vi "FW_readFiles.vi"(4 "frame_offset":i32, 6 "amount_frames":u32, 7 "Decimate_frameRate":i32, 8 "error in (no error)":errorcluster, 10 "path(dir/img)":path[](array[path]), 11 "JPG/AVI (F:JPG)":bool) -> (0 "error out":errorcluster, 2 "image_path_array_out":path[](array[path]), 3 "image_array_out":T1[](array[typedef]), 5 "root folder":path)   [LabVIEW 2021, in "Framework_lib.lvlib"]
uses:
  QMH/Framework_lib.lvlib
  <vilib>/vision/Image Controls.llb/IMAQ Image.ctl
  <vilib>/vision/Avi.llb/IMAQ AVI2 Codec Path.ctl
panel:
  out "frame #":i32
  out "elapsed(ms)":u32
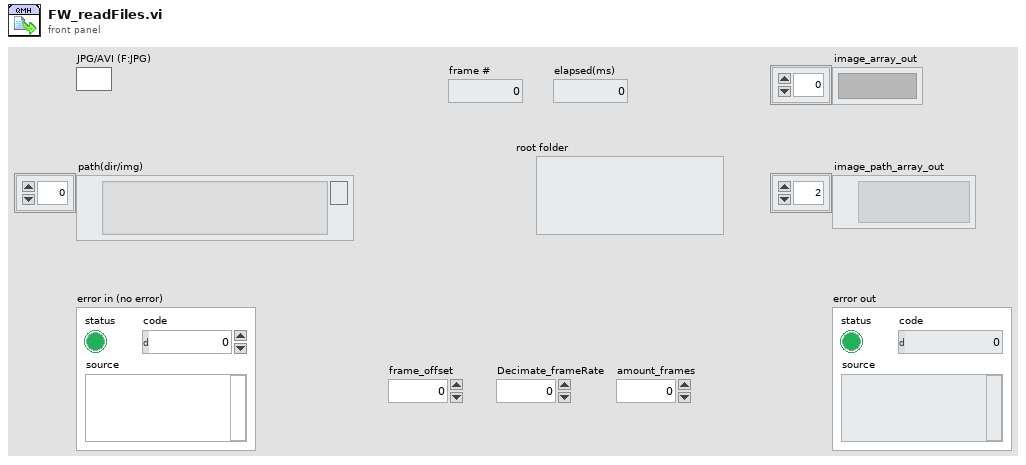
[diagram p1: front panel]
types:
  T1 = typedef "IMAQ Image.ctl" = refnum<image>
  T2 = typedef "IMAQ AVI2 Codec Path.ctl" = u32
  T3 = typedef "IMAQ AVI2 Refnum.ctl" = refnum<k20>
  T4 = typedef "Image Type" = u32
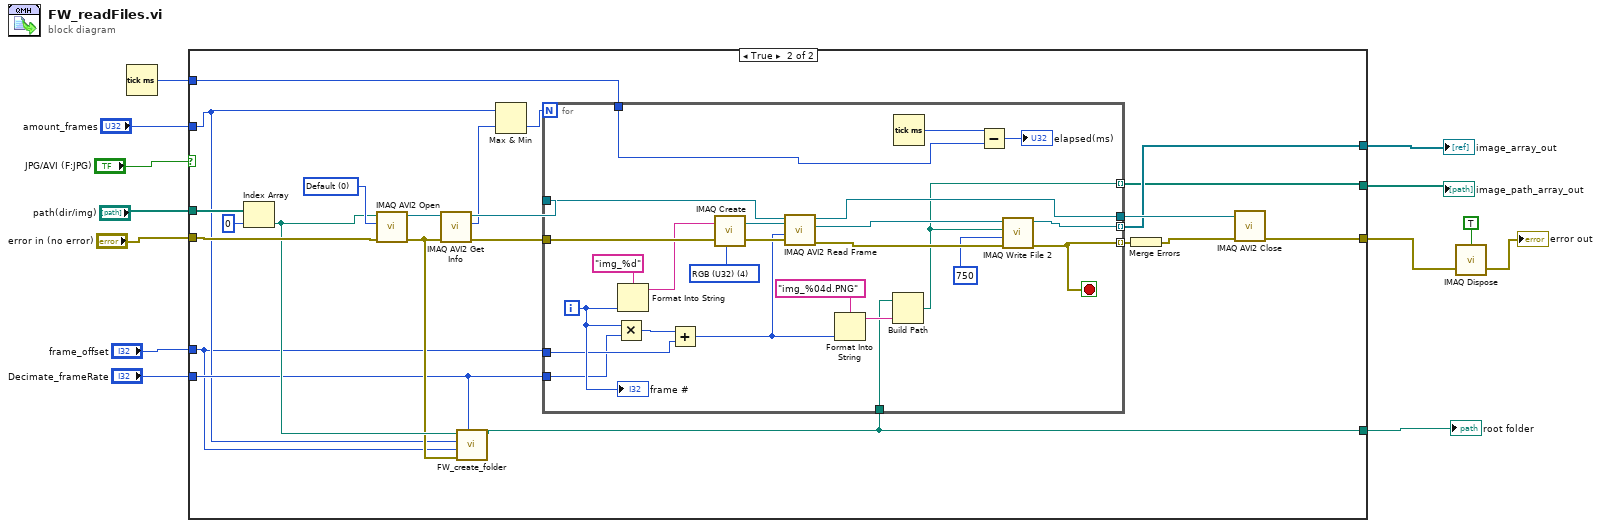
[diagram p0: block diagram]
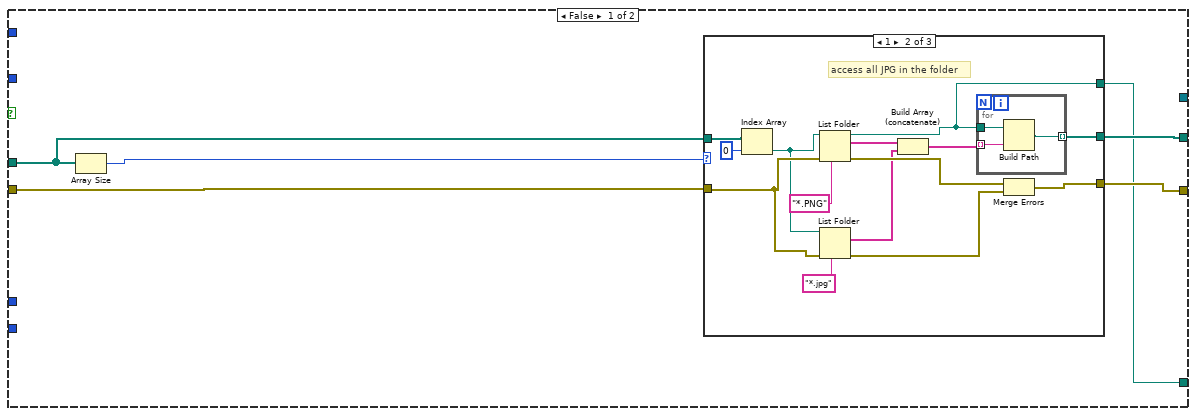
[diagram p2: hidden frame]
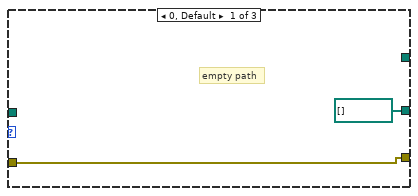
[diagram p3: hidden frame]
diagram:
  n1 = Tick Count (ms)() -> (millisecond timer value=w4:u32)
  n2 = case shown="True" "JPG/AVI (F:JPG)" {
    tunnel: "path(dir/img)" -> [w18 w61]
    tunnel: "error in (no error)" -> [w17 w59]
    tunnel: [w16 w58] -> w13
    tunnel: [w15 w46] -> w9
    tunnel: [_ w51] -> w8
    tunnel: "amount_frames" -> [_ w42]
    tunnel: "frame_offset" -> [_ w41]
    tunnel: "Decimate_frameRate" -> [_ w45]
    tunnel: w4 -> [_ w44]
    tunnel: [w14 w43] -> w3
    frame False {
      n3 = Array Size(array=w18) -> (size(s)=w19:i32)
      n4 = case shown="1" w19 {
        tunnel: w18 -> [_ w35 w40]
        tunnel: w17 -> [w20 w27 w39]
        tunnel: [w20 w26 w39] -> w16
        tunnel: [path[] [] w30 w40] -> w15
        tunnel: [_ w29 _] -> w14
        frame 0, Default {
          # "empty path"
        }
        frame 1 {
          # "access all JPG in the folder"
          n5 = Index Array(array=w35, index=0) -> (element=w22:path)
          n6 = List Folder(path=w22, pattern="*.PNG", error in=w27) -> (path out=w29:path, filenames=w31:string[], error out=w32:errorcluster)  [unwired: 1 in, 1 out]
          n7 = List Folder(path=w22, pattern="*.jpg", error in=w27) -> (filenames=w23:string[], error out=w25:errorcluster)  [unwired: 1 in, 2 out]
          n8 = Build Array (concatenate)(w31, w23) -> (w24:string[])
          n9 = for {
            tunnel: w29 -> [w38]
            tunnel: w24 -> [w37] mode=indexing
            tunnel: [w36] -> w30 mode=indexing
            n10 = Build Path(base path=w38, name or relative path=w37) -> (appended path=w36:path)
          }
          n11 = Merge Errors(w32, w25) -> (w26:errorcluster)
        }
        frame 2.. {
          # "read each file (must be JPG)"
        }
      }
    }
    frame True {
      w62 = T2 0 items=["Default", "System", "Built in Vision"] ("Codec Source")
      n12 = Index Array(array=w61, index=0) -> (element=w48:path)
      n13 = call "IMAQ AVI2 Open"("error in (no error)"=w59, "Codec Source"=w62, "AVI File Path"=w48) -> ("error out"=w47:errorcluster, "AVI Refnum"=w57:T3)  [unwired: 7 in]
      n14 = call "IMAQ AVI2 Get Info"("error in (no error)"=w47, "AVI Refnum"=w57) -> ("error out"=w56:errorcluster, "Number of Frames"=w50:u32, "AVI Refnum (duplicate)"=w55:T3)  [unwired: 5 in, 2 out]
      n15 = call "FW_create_folder.vi"("Decimate_frameRate"=w45, "error in (no error)"=w47, "frame_offset"=w41, "amount_frames"=w42, "Path"=w48) -> ("created path"=w43:path)  [unwired: 5 in, 1 out]
      n16 = Max & Min(x=w42, y=w50) -> (min(x,y)=w49:u32)  [unwired: 1 out]
      n17 = for {
        N: w49 -> [_]
        tunnel: w56 -> [w87]
        tunnel: w55 -> [w83]
        tunnel: [w77] -> w54 mode=indexing
        tunnel: [w81] -> w53
        tunnel: [w75] -> w51 mode=indexing
        tunnel: w41 -> [w74]
        tunnel: w43 -> [w71]
        tunnel: [w70] -> w46 mode=indexing
        tunnel: w45 -> [w68]
        tunnel: w44 -> [w64]
        i -> [w78]
        stop <- w77 stop-if-true
        w86 = T4 4 items=["Grayscale (U8)", "Grayscale (I16)", "Grayscale (SGL)", "Complex (CSG)", "RGB (U32)", "HSL (U32)", "RGB (U64)", "Grayscale (U16)"] ("Image Type")
        n18 = Multiply(x=w78, y=w68) -> (x*y=w69:i32)
        n19 = Format Into String(format string="img_%d", w78) -> (resulting string=w80:string)  [unwired: 2 in, 1 out]
        n20 = Add(x=w69, y=w74) -> (x+y=w67:i32)
        n21 = call "IMAQ Create"("Image Name"=w80, "Image Type"=w86, "error in (no error)"=w87) -> ("New Image"=w84:T1, "error out"=w85:errorcluster)  [unwired: 2 in]
        n22 = call "IMAQ AVI2 Read Frame"("error in (no error)"=w85, "Frame Number"=w67, "Image"=w84, "AVI Refnum"=w83) -> ("error out"=w82:errorcluster, "Image Out"=w76:T1, "AVI Refnum (duplicate)"=w81:T3)  [unwired: 5 in]
        n23 = Format Into String(format string="img_%04d.PNG", w67) -> (resulting string=w72:string)  [unwired: 2 in, 1 out]
        n24 = Build Path(base path=w71, name or relative path=w72) -> (appended path=w70:path)
        n25 = Tick Count (ms)() -> (millisecond timer value=w65:u32)
        n26 = Subtract(x=w65, y=w64) -> (x-y=→"elapsed(ms)":u32)
        n27 = call-poly "IMAQ Write File 2"("error in (no error)"=w82, "Image Quality"=u32 750, "File Path"=w70, "Image"=w76) -> ("error out"=w77:errorcluster, "Image Out (duplicate)"=w75:T1)  [unwired: 6 in]
        "frame #" <- w78
      }
      n28 = Merge Errors(w54) -> (w52:errorcluster)
      n29 = call "IMAQ AVI2 Close"("error in (no error)"=w52, "AVI Refnum"=w53) -> ("error out"=w58:errorcluster)  [unwired: 9 in]
    }
  }
  "image_path_array_out" <- w9
  "image_array_out" <- w8
  "root folder" <- w3
  n30 = call "IMAQ Dispose"("All Images? (No)"=TRUE, "error in (no error)"=w13) -> ("error out"=→"error out":errorcluster)  [unwired: 4 in]
